vi "Initiate Acquisition.vi"(8 "error in (no error)":errorcluster, 11 "CS++Scope":refnum<class "CS++Scope.lvclass">) -> (0 "error out":errorcluster, 3 "CS++Scope out":refnum<class "CS++Scope.lvclass">)   [LabVIEW 2014, in "CS++Scope.lvlib" / "CS++Scope.lvclass"]
doc: "This VI initiates a waveform acquisition. After you call this VI, the oscilloscope leaves the Idle state and waits for a trigger. The oscilloscope acquires a waveform for each channel you have enabled with the IviScope Configure Channel VI.\n\nNote (1) This VI does not check the instrument status. Typically, you call this VI only in a sequence of calls to other low-level driver VIs. The sequence performs one operation. You use the low-level VIs to optimize one or more aspects of interaction with the instrument. If you want to check the instrument status, call the IviScope Error-Query VI at the conclusion of the sequence.\n(2) This VI performs interchangeability checking when the IviScope>>Inherent IVI Settings>>User Options>>Interchange Check property is set to TRUE. If the IviScope>>Inherent IVI Settings>>User Options>>Spy property is set to TRUE, you use the NI I/O Trace utility to view interchangeability warnings. You use the IviScope Get Next Interchange Warning VI to retrieve interchangeability warnings when the IviScope>>Inherent IVI Settings>>User Options>>Spy property is set to FALSE. For more information about interchangeability checking, refer to the help text for the IviScope>>Inherent IVI Settings>>User Options>>Interchange Check property.\n(3) The class driver performs a simulated waveform acquisition when this VI is called and the IviScope>>Inherent IVI Settings>>User Options>>Simulate property is set to TRUE and the IviScope>>Inherent IVI Settings>>User Options>>Use Specific Simulation property is set to FALSE. For information on how to configure a simulated waveform, refer to the online help manual."
uses:
  CS++Scope.lvclass
  CS++Scope.lvclass/CS++Scope.ctl
  <vilib>/ActorFramework/Actor/Actor.lvclass/Actor.ctl
  <vilib>/ActorFramework/Message Enqueuer/Message Enqueuer.lvclass/Message Enqueuer.ctl
  CS++Scope Messages/Fetch Waveform Msg/Fetch Waveform Msg.lvclass/Fetch Waveform Msg.ctl
  <vilib>/ActorFramework/Message Enqueuer/Init from Existing Queue.vi
  <vilib>/ActorFramework/Message Enqueuer/Enqueue.vi
  <vilib>/ActorFramework/Message Priority Queue/Priority Enqueue.vi
  <vilib>/ActorFramework/Message Enqueuer/Message Enqueuer.lvclass
  CS++Scope Messages/Fetch Waveform Msg/Fetch Waveform Msg.lvclass
  <vilib>/ActorFramework/Actor/Actor.lvclass
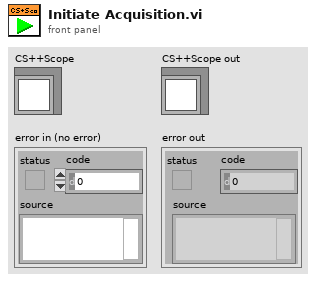
[diagram p1: front panel]
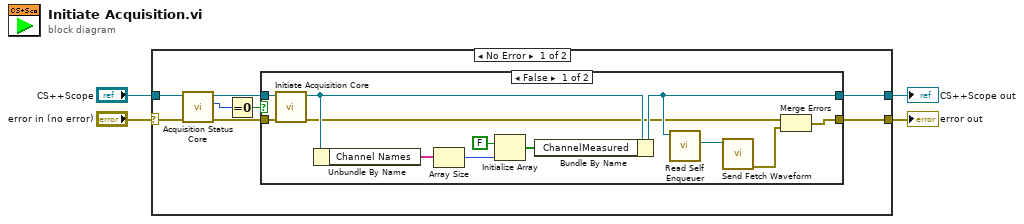
[diagram p0: block diagram]
diagram:
  n1 = case shown="No Error" "error in (no error)" {
    selector: "error in (no error)" -> [w9 w28]
    tunnel: [w6 w28] -> w3
    tunnel: [w12 w27] -> w2
    tunnel: "CS++Scope" -> [w11 w27]
    frame No Error {
      n2 = call-dynamic "Acquisition Status Core.vi"("error in (no error)"=w9, "CS++Scope"=w11) -> ("error out"=w8:errorcluster, "acquisition status"=w7:i32, "CS++Scope out"=w10:refnum<class "CS++Scope.lvclass">)  [unwired: 7 in]
      n3 = Equal To 0?(x=w7) -> (x = 0?=w5:bool)
      n4 = case shown="False" w5 {
        tunnel: [w16 w25] -> w12
        tunnel: w10 -> [w23 w25]
        tunnel: w8 -> [w22 w26]
        tunnel: [w13 w26] -> w6
        frame False {
          n5 = call-dynamic "Initiate Acquisition Core.vi"("error in (no error)"=w22, "CS++Scope"=w23) -> ("error out"=w14:errorcluster, "CS++Scope out"=w24:refnum<class "CS++Scope.lvclass">)  [unwired: 8 in]
          n6 = Unbundle By Name(w24) -> ("Channel Names"=w21:string[])
          n7 = Array Size(array=w21) -> (size(s)=w20:i32)
          n8 = Initialize Array(FALSE, w20) -> (w18:bool[])
          n9 = Bundle By Name(cluster=w24, "ChannelMeasured"=w18) -> (w16:refnum<class "CS++Scope.lvclass">)
          n10 = call <vilib>:"Read Self Enqueuer.vi"("Actor"=w16) -> ("Self Enqueuer"=w17:refnum<class "Message Enqueuer.lvclass">)  [unwired: 10 in]
          n11 = call "Send Fetch Waveform.vi"("Message Enqueuer"=w17) -> ("error out"=w15:errorcluster)  [unwired: 9 in, 1 out]
          n12 = Merge Errors(w14, w15) -> (w13:errorcluster)
        }
        frame True {
        }
      }
    }
    frame Error {
    }
  }
  "error out" <- w3
  "CS++Scope out" <- w2
